vi "Error_Control.vi"(2 "Command (Handle Errors)":T1=enum."Handle Errors", 5 "Test Loop":refnum<queue>, 7 "UI Loop Error":refnum<user-event>, 11 "Error In":errorcluster) -> (15 "Error Out":errorcluster)   [LabVIEW 2016]
doc: "This VI performs the error handling and reporting for the application. If an error occurs it will send Queues and Error User Events to the different loops to shutdown the application."
uses:
  controls/Error_Command.ctl
  controls/states.ctl
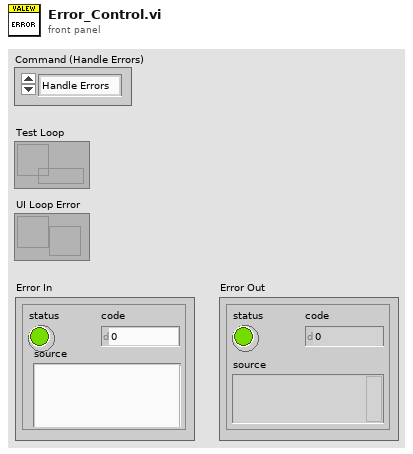
[diagram p1: front panel]
types:
  T1 = typedef "Error_Command.ctl" = enum16{"Initialize", "Handle Errors", "Report Errors"}
  T2 = typedef "states.ctl" = enum16{"Wait for Barcode Scan", "Confirm Board Setup", "Initialization", "Perosnality Test", "Button Test", "LED Test", "ADC Knob Test", "Pressure Sensor Test", "Test Complete", "Log Results", "Re-Init Test", "Shutdown"}
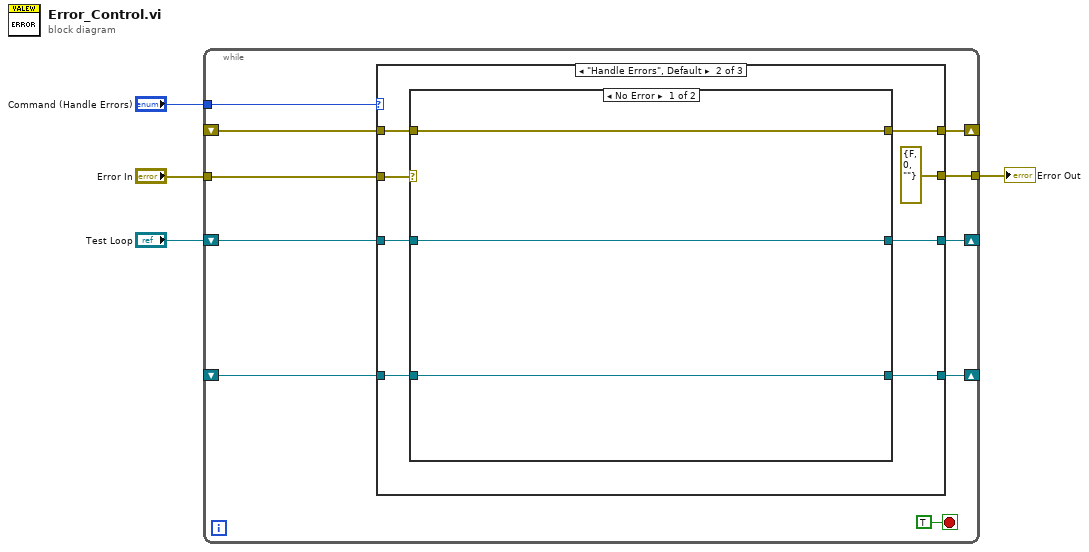
[diagram p0: block diagram]
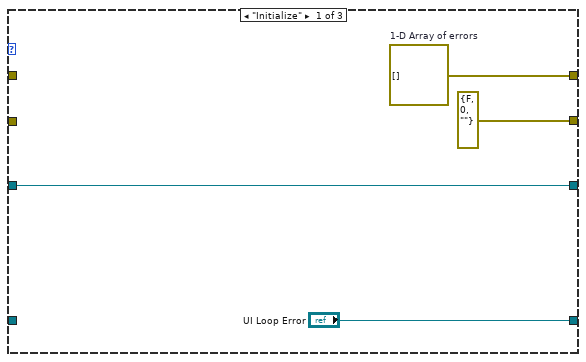
[diagram p2: hidden frame]
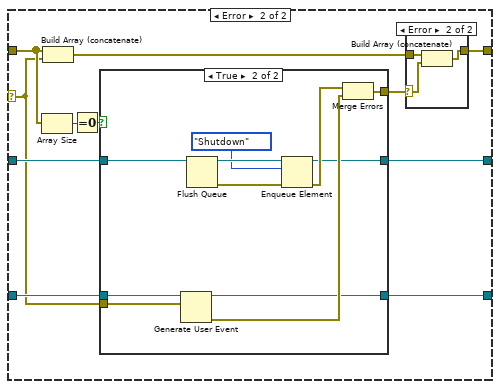
[diagram p3: hidden frame]
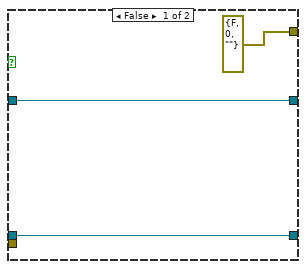
[diagram p4: hidden frame]
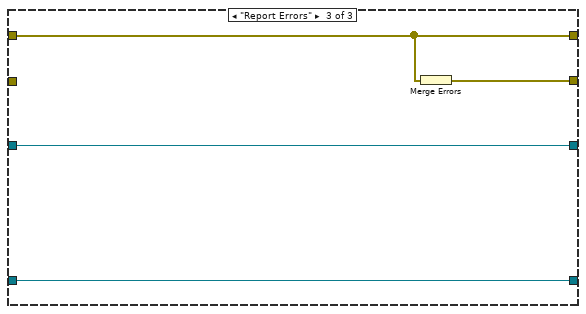
[diagram p6: hidden frame]
diagram:
  n1 = while {
    tunnel: "Error In" -> [w12]
    tunnel: "Command (Handle Errors)" -> [w13]
    shift-right: [w11] -> _
    shift-left: _ -> [w10]
    tunnel: [w9] -> w2
    shift-right: [w8] -> _
    shift-left: "Test Loop" -> [w7]
    shift-right: [w5] -> _
    shift-left: _ -> [w6]
    stop <- TRUE stop-if-true
    n2 = case shown="\"Handle Errors\", Default" w13 {
      tunnel: w12 -> [_ w26 _]
      tunnel: [w18 w22 w61] -> w11
      tunnel: w10 -> [_ w25 w61]
      tunnel: [errorcluster {"status"=FALSE, "code"=0, "source"=""} ("Error In") errorcluster {"status"=FALSE, "code"=0, "source"=""} ("Error In") w62] -> w9
      tunnel: [w16 w21 w60] -> w8
      tunnel: w7 -> [w16 w24 w60]
      tunnel: w6 -> [_ w23 w59]
      tunnel: ["UI Loop Error" w19 w59] -> w5
      frame "Initialize" {
        w18 = errorcluster[] []  # 1-D Array of errors
      }
      frame "Handle Errors", Default {
        n3 = case shown="No Error" w26 {
          selector: w26 -> [_ w33]
          tunnel: w25 -> [w29 w40]
          tunnel: w24 -> [w28 w37]
          tunnel: w23 -> [w27 w36]
          tunnel: [w29 w34] -> w22
          tunnel: [w28 w32] -> w21
          tunnel: [w27 w30] -> w19
          frame No Error {
          }
          frame Error {
            n4 = Array Size(array=w40) -> (size(s)=w39:i32)
            n5 = Build Array (concatenate)(w40, w33) -> (w31:errorcluster[])
            n6 = Equal To 0?(x=w39) -> (x = 0?=w38:bool)
            n7 = case shown="True" w38 {
              tunnel: w37 -> [w42 w54]
              tunnel: w36 -> [w41 w45]
              tunnel: [errorcluster {"status"=FALSE, "code"=0, "source"=""} ("error IO") w53] -> w35
              tunnel: w33 -> [_ w50]
              tunnel: [w42 w47] -> w32
              tunnel: [w41 w44] -> w30
              frame False {
              }
              frame True {
                n8 = Generate User Event(user event=w45, event data cluster=w50) -> (user event out=w44:refnum<user-event>, error out=w49:errorcluster)  [unwired: 2 in]
                n9 = Flush Queue(queue=w54) -> (queue out=w51:refnum<queue>, error out=w52:errorcluster)  [unwired: 1 in, 1 out]
                n10 = Enqueue Element(queue=w51, element=states."Shutdown" ("Enum"), error in (no error)=w52) -> (queue out=w47:refnum<queue>, error out=w48:errorcluster)  [unwired: 1 in, 1 out]
                n11 = Merge Errors(w48, w49) -> (w53:errorcluster)
              }
            }
            n12 = case shown="Error" w35 {
              selector: w35 -> [_ w57]
              tunnel: [w55 w58] -> w34
              tunnel: w31 -> [w55 w56]
              frame No Error {
              }
              frame Error {
                n13 = Build Array (concatenate)(w56, w57) -> (w58:errorcluster[])
              }
            }
          }
        }
      }
      frame "Report Errors" {
        n14 = Merge Errors(w61) -> (w62:errorcluster)
      }
    }
  }
  "Error Out" <- w2
